vi "LWXPS_PositionerCorrectorPIDBaseSet.vi"(0 "Positioner Name":string, 1 "XPS Reference IN":refnum<k24>, 5 "Moving Mass":dbl, 7 "Static Mass":dbl, 9 "Viscosity":dbl, 11 "Stiffness":dbl, 12 "LabVIEW error IN":errorcluster) -> (4 "XPS Reference OUT":refnum<k24>, 6 "Returned error code":i32, 10 "XPS Error String":string, 15 "LabVIEW error OUT":errorcluster)   [LabVIEW 2014]
uses:
  D:/XPSQ8_LabView_Library/Development/Source/Dll/Newport.XPS.CommandInterface.dll
  Dll/Newport.XPS.CommandInterface.dll
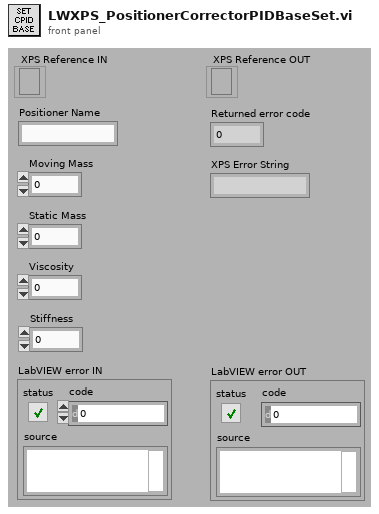
[diagram p1: front panel]
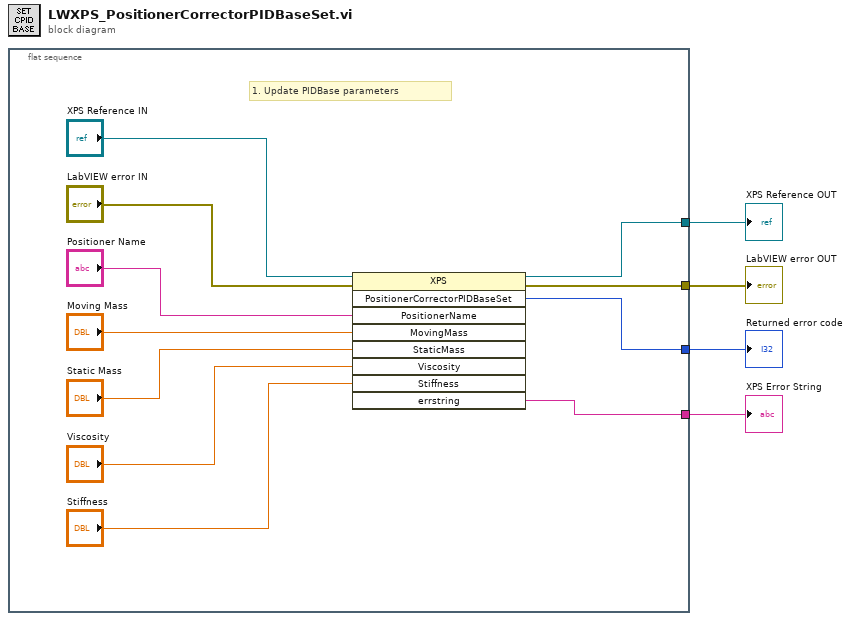
[diagram p0: block diagram]
diagram:
  n1 = flat-sequence {
    tunnel: [w11] -> w4
    tunnel: [w10] -> w3
    tunnel: [w12] -> w2
    tunnel: [w6] -> w1
    frame #0 {
      # "1. Update PIDBase parameters"
      n2 = invoke class="XPS" method="PositionerCorrectorPIDBaseSet"(reference="XPS Reference IN", error in="LabVIEW error IN", "PositionerName"="Positioner Name", "MovingMass"="Moving Mass", "StaticMass"="Static Mass", "Viscosity"="Viscosity", "Stiffness"="Stiffness") -> (reference out=w11:refnum<k24>, error out=w10:errorcluster, "PositionerCorrectorPIDBaseSet"=w12:i32, "errstring"=w6:string)  [unwired: 2 in, 5 out]
    }
  }
  "XPS Error String" <- w1
  "XPS Reference OUT" <- w4
  "LabVIEW error OUT" <- w3
  "Returned error code" <- w2
